vi "F Dwf Analog Out Node Phase Set.vi"(7 "degreePhase":dbl, 8 "error in (no error)":errorcluster, 9 "node":i32, 10 "idxChannel":i32, 11 "hdwf":i32) -> (0 "error out":errorcluster, 3 "function return":i32)   [LabVIEW 2024, in "Olasdwf.lvlib"]
doc: "DWFAPI int FDwfAnalogOutNodePhaseSet(HDWF hdwf, int idxChannel, AnalogOutNode node, double degreePhase);"
uses:
  Olasdwf.lvlib
  Windows/System32/dwf.dll
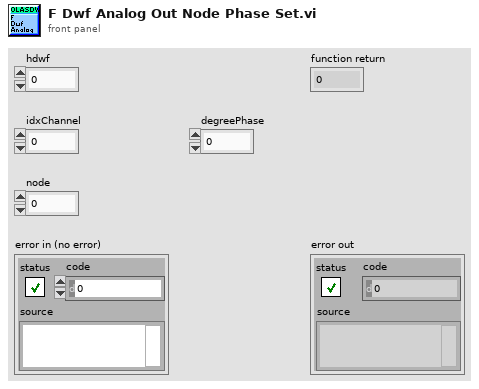
[diagram p1: front panel]
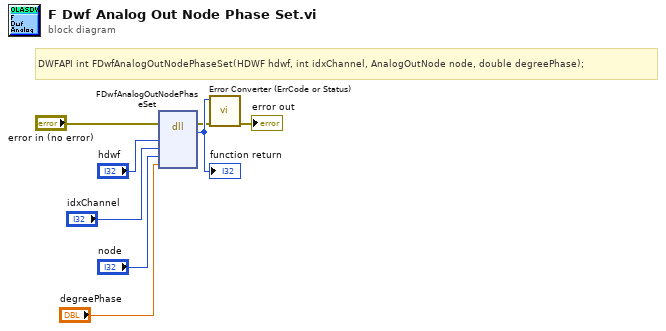
[diagram p0: block diagram]
diagram:
  # "DWFAPI int FDwfAnalogOutNodePhaseSet(HDWF hdwf, int idxChannel, AnalogOutNode node, double degreePhase);"
  n1 = dll-call lib="/Windows/System32/dwf.*" fn="FDwfAnalogOutNodePhaseSet"(error in="error in (no error)", "hdwf"="hdwf", "idxChannel"="idxChannel", "node"="node", "degreePhase"="degreePhase") -> (error out=w2:errorcluster, w8:i32)  [unwired: 6 in, 1 out]
  "function return" <- w8
  n2 = call "Error Converter (ErrCode or Status).vi"("error in (no error)"=w2, "error code"=w8) -> ("error out"=→"error out":errorcluster)  [unwired: 9 in]
